vi "GPS Navigation & Obstacle Avoidance.vi"   [LabVIEW 2011]
uses:
  _GlobalVariables&Libraries/ATV Program Global Variables.vi
types:
  T1 = cluster{"End ATV Program":bool, "E-Stop":bool, "Save Logfile":bool, "Logfile Iteration Delay (ms)":u32, "Loop iteration time (ms)":u32, "Logfile Location":path, "Default GPS Navigation Path":path, "Computer":string, "Default GPS Boundary Path":path}
  T2 = cluster{"Navigation Coordinates":cluster{"Latitude":dbl, "Longitude":dbl}[], "Coordinate Count":u32, "Drive Speed":string, "Steer Angle":dbl, "Steering":dbl, "Direction to next Coordinate":dbl, "Drive":dbl, "Navigation Path":string}
  T3 = cluster{"Drive Value Output String":string, "Steer Value Output String":string, "Button A":bool, "Button B":bool, "Error Out":errorcluster, "Disable XBox Drive & Steer":bool, "Disable XBox Controller":bool, "XBOX Button Trigger Time (ms)":u32, "Button X":bool, "Button Y":bool}
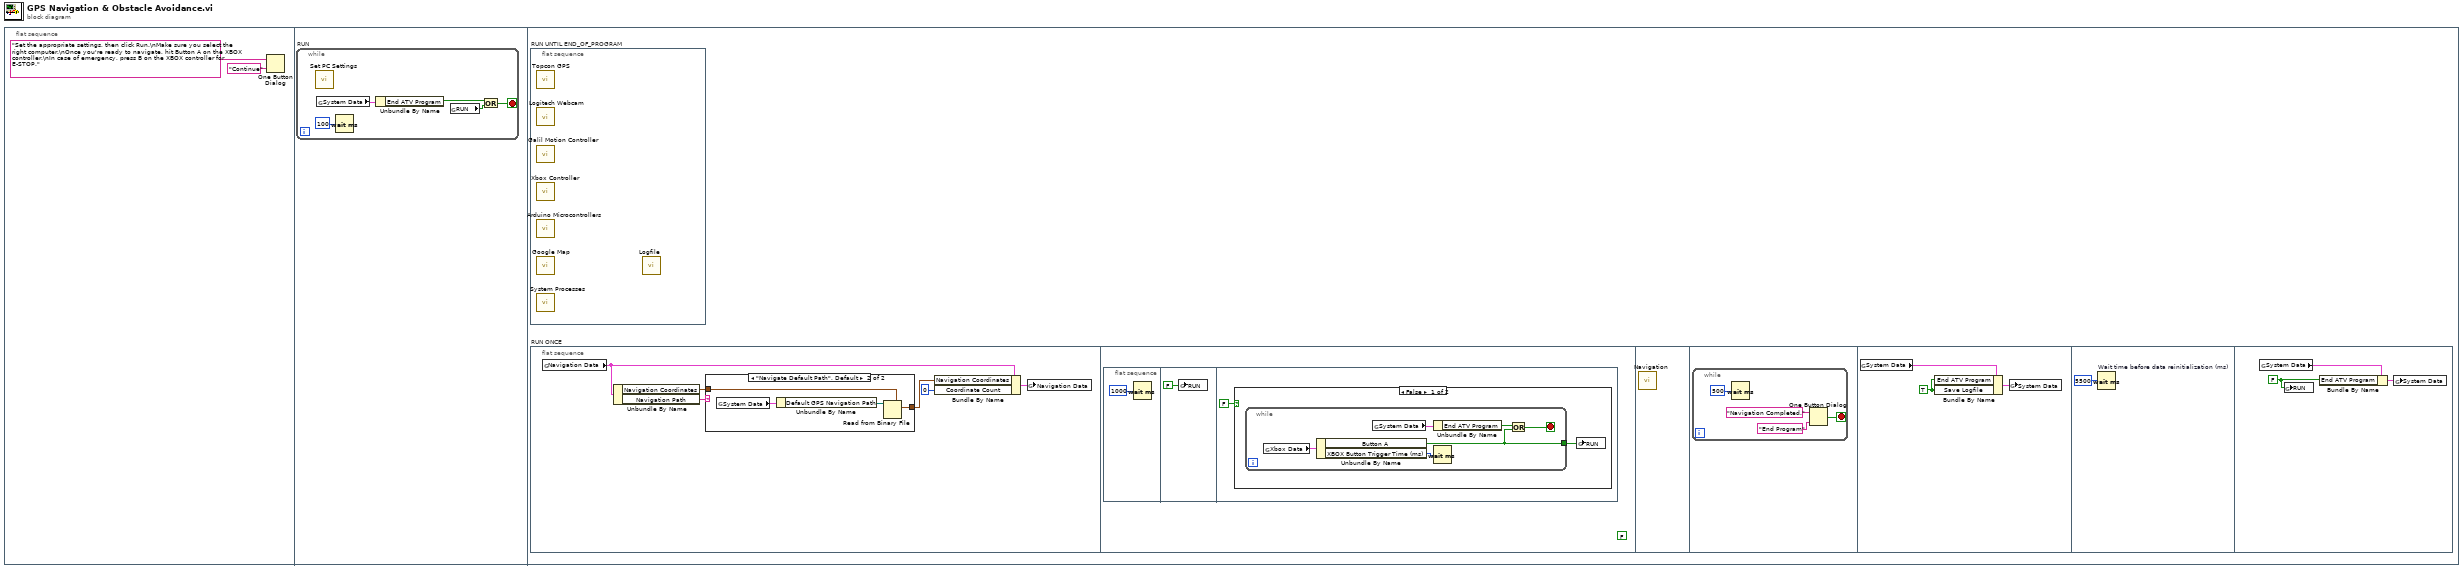
[diagram p0: block diagram]
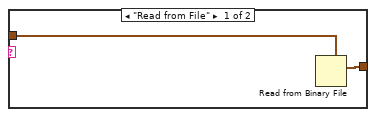
[diagram p2: hidden frame]
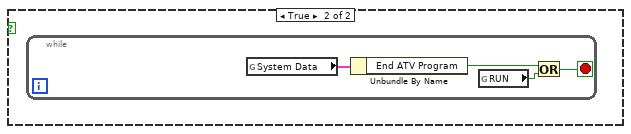
[diagram p3: hidden frame]
diagram:
  n1 = flat-sequence {
    frame #0 {
      n2 = One Button Dialog(message="Set the appropriate settings, then click Run.\nMake sure you select the right computer.\nOnce you're ready to navigate, hit Button A on the XBOX controller.\nIn case of emergency, press B on the XBOX controller for E-STOP.", button name ("OK")="Continue") -> ()  [unwired: 1 out]
    }
    frame #1 {
      n3 = while "RUN" {
        stop <- w3 stop-if-true
        n4 = call "Set PC Settings.vi"() -> ()  [unwired: 12 in]
        n5 = global read "ATV Program Global Variables.vi" "System Data"() -> (w6:T1)
        n6 = Wait (ms)(milliseconds to wait=u32 100) -> ()  [unwired: 1 out]
        n7 = Unbundle By Name(w6) -> ("End ATV Program"=w4:bool)
        n8 = global read "ATV Program Global Variables.vi" "RUN"() -> (w5:bool)
        n9 = Or(x=w4, y=w5) -> (x .or. y?=w3:bool)
      }
    }
    frame #2 {
      n10 = flat-sequence "RUN UNTIL END_OF_PROGRAM" {
        frame #0 {
          n11 = call "Topcon GPS.vi"() -> ()  [unwired: 12 in]
          n12 = call "Logitech Webcam.vi"() -> ()  [unwired: 12 in]
          n13 = call "Galil Motion Controller.vi"() -> ()  [unwired: 1 in]
          n14 = call "Xbox Controller.vi"() -> ()  [unwired: 1 in]
          n15 = call "Arduino Microcontrollers.vi"() -> ()  [unwired: 1 in]
          n16 = call "Google Map.vi"() -> ()  [unwired: 1 in]
          n17 = call "System Processes.vi"() -> ()  [unwired: 12 in]
          n18 = call "Logfile.vi"() -> ()  [unwired: 12 in]
        }
      }
      n19 = flat-sequence "RUN ONCE" {
        frame #0 {
          n20 = global read "ATV Program Global Variables.vi" "Navigation Data"() -> (w13:T2)
          n21 = Unbundle By Name(w13) -> ("Navigation Coordinates"=w8:cluster{"Latitude":dbl, "Longitude":dbl}[], "Navigation Path"=w10:string)
          n22 = case shown="\"Navigate Default Path\", Default" w10 {
            tunnel: [w14 w18] -> w9
            tunnel: w8 -> [w15 w17]
            frame "Read from File" {
              n23 = Read from Binary File(5:w15) -> (2:w14:cluster{"Latitude":dbl, "Longitude":dbl}[])  [unwired: 5 in, 3 out]
            }
            frame "Navigate Default Path", Default {
              n24 = global read "ATV Program Global Variables.vi" "System Data"() -> (w19:T1)
              n25 = Unbundle By Name(w19) -> ("Default GPS Navigation Path"=w16:path)
              n26 = Read from Binary File(5:w17, 11:w16) -> (2:w18:cluster{"Latitude":dbl, "Longitude":dbl}[])  [unwired: 4 in, 3 out]
            }
          }
          n27 = Bundle By Name(cluster=w13, "Navigation Coordinates"=w9, "Coordinate Count"=u32 0) -> (w12:T2)
          n28 = global write "ATV Program Global Variables.vi" "Navigation Data"(w12) -> ()
        }
        frame #1 {
          (unwired) FALSE
          n29 = flat-sequence {
            frame #0 {
              n30 = Wait (ms)(milliseconds to wait=u32 1000) -> ()  [unwired: 1 out]
            }
            frame #1 {
              n31 = global write "ATV Program Global Variables.vi" "RUN"(FALSE ("RUN")) -> ()
            }
            frame #2 {
              n32 = case shown="False" FALSE {
                frame False {
                  n33 = while {
                    tunnel: [w25] -> w23
                    stop <- w24 stop-if-true
                    n34 = global read "ATV Program Global Variables.vi" "Xbox Data"() -> (w29:T3)
                    n35 = Unbundle By Name(w29) -> ("Button A"=w25:bool, "XBOX Button Trigger Time (ms)"=w28:u32)
                    n36 = global read "ATV Program Global Variables.vi" "System Data"() -> (w27:T1)
                    n37 = Unbundle By Name(w27) -> ("End ATV Program"=w26:bool)
                    n38 = Wait (ms)(milliseconds to wait=w28) -> ()  [unwired: 1 out]
                    n39 = Or(x=w26, y=w25) -> (x .or. y?=w24:bool)
                  }
                  n40 = global write "ATV Program Global Variables.vi" "RUN"(w23) -> ()
                }
                frame True {
                  n41 = while {
                    stop <- w30 stop-if-true
                    n42 = global read "ATV Program Global Variables.vi" "System Data"() -> (w33:T1)
                    n43 = Unbundle By Name(w33) -> ("End ATV Program"=w32:bool)
                    n44 = global read "ATV Program Global Variables.vi" "RUN"() -> (w31:bool)
                    n45 = Or(x=w32, y=w31) -> (x .or. y?=w30:bool)
                  }
                }
              }
            }
          }
        }
        frame #2 {
          n46 = call "Navigation.vi"() -> ()  [unwired: 1 in]
        }
        frame #3 {
          n47 = while {
            stop <- w34 stop-if-true
            n48 = Wait (ms)(milliseconds to wait=u32 500) -> ()  [unwired: 1 out]
            n49 = One Button Dialog(message="Navigation Completed.", button name ("OK")="End Program") -> (true=w34:bool)
          }
        }
        frame #4 {
          w38 = TRUE ("End Program")
          n50 = global read "ATV Program Global Variables.vi" "System Data"() -> (w40:T1)
          n51 = Bundle By Name(cluster=w40, "End ATV Program"=w38, "Save Logfile"=w38) -> (w39:T1)
          n52 = global write "ATV Program Global Variables.vi" "System Data"(w39) -> ()
        }
        frame #5 {
          n53 = Wait (ms) "Wait time before data reinitialization (ms)"(milliseconds to wait=u32 5500) -> ()  [unwired: 1 out]
        }
        frame #6 {
          w42 = FALSE ("End Program")
          n54 = global read "ATV Program Global Variables.vi" "System Data"() -> (w43:T1)
          n55 = global write "ATV Program Global Variables.vi" "RUN"(w42) -> ()
          n56 = Bundle By Name(cluster=w43, "End ATV Program"=w42) -> (w44:T1)
          n57 = global write "ATV Program Global Variables.vi" "System Data"(w44) -> ()
        }
      }
    }
  }
